vi "Save Digital Patterns.vi"(8 "error in (no error)":errorcluster, 10 "Patterns":T1[](array[typedef]), 11 "Item Ref in":T5 format="%.0x") -> (0 "error out":errorcluster)   [LabVIEW 2019, in "Engine Simulation Toolkit System Explorer.lvlib"]
uses:
  Engine Simulation Toolkit System Explorer.lvlib
  <vilib>/NI VeriStand/Custom Device API/Custom Device Item Ref.ctl
  Digital Pattern.ctl
  Digital Pattern Base.ctl
  Digital Pattern Remove Edge.ctl
  Digital Pattern Add Pulse.ctl
  Shared/Properties.vi
  <vilib>/NI VeriStand/Custom Device API/Set Item Property (String).vi
  <vilib>/NI VeriStand/Custom Device API/Set Item Property (Double).vi
  <vilib>/NI VeriStand/Custom Device API/Set Item Property (U16).vi
  <vilib>/NI VeriStand/Custom Device API/Set Item Property (Boolean).vi
  Shared/Engine Simulation Toolkit Shared.lvlib
  <vilib>/NI VeriStand/Custom Device API/Custom Device API.lvlib
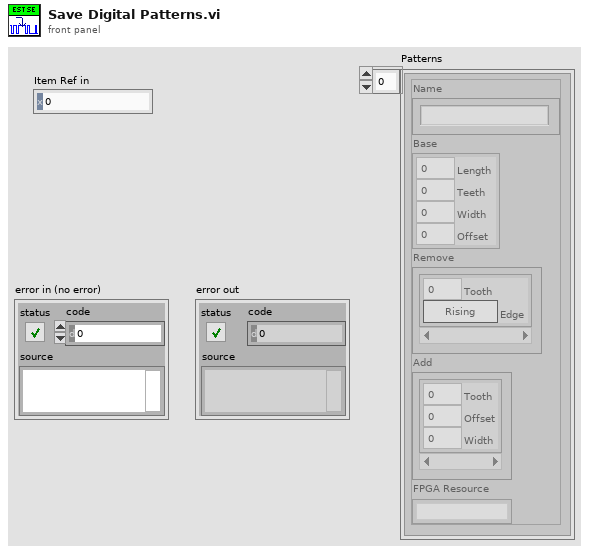
[diagram p1: front panel]
types:
  T1 = typedef "Engine Simulation Toolkit System Explorer.lvlib/Digital Pattern.ctl" = cluster{"Name":string, "Base":T2, "Remove":T3[], "Add":T4[], "FPGA Resource":string}
  T2 = typedef "Engine Simulation Toolkit System Explorer.lvlib/Digital Pattern Base.ctl" = cluster{"Length":dbl, "Teeth":u16, "Width":dbl, "Offset":dbl}
  T3 = typedef "Engine Simulation Toolkit System Explorer.lvlib/Digital Pattern Remove Edge.ctl" = cluster{"Tooth":u16, "Edge":bool}
  T4 = typedef "Engine Simulation Toolkit System Explorer.lvlib/Digital Pattern Add Pulse.ctl" = cluster{"Tooth":u16, "Offset":dbl, "Width":dbl}
  T5 = typedef "Custom Device API.lvlib/Custom Device Item Ref.ctl" = u64
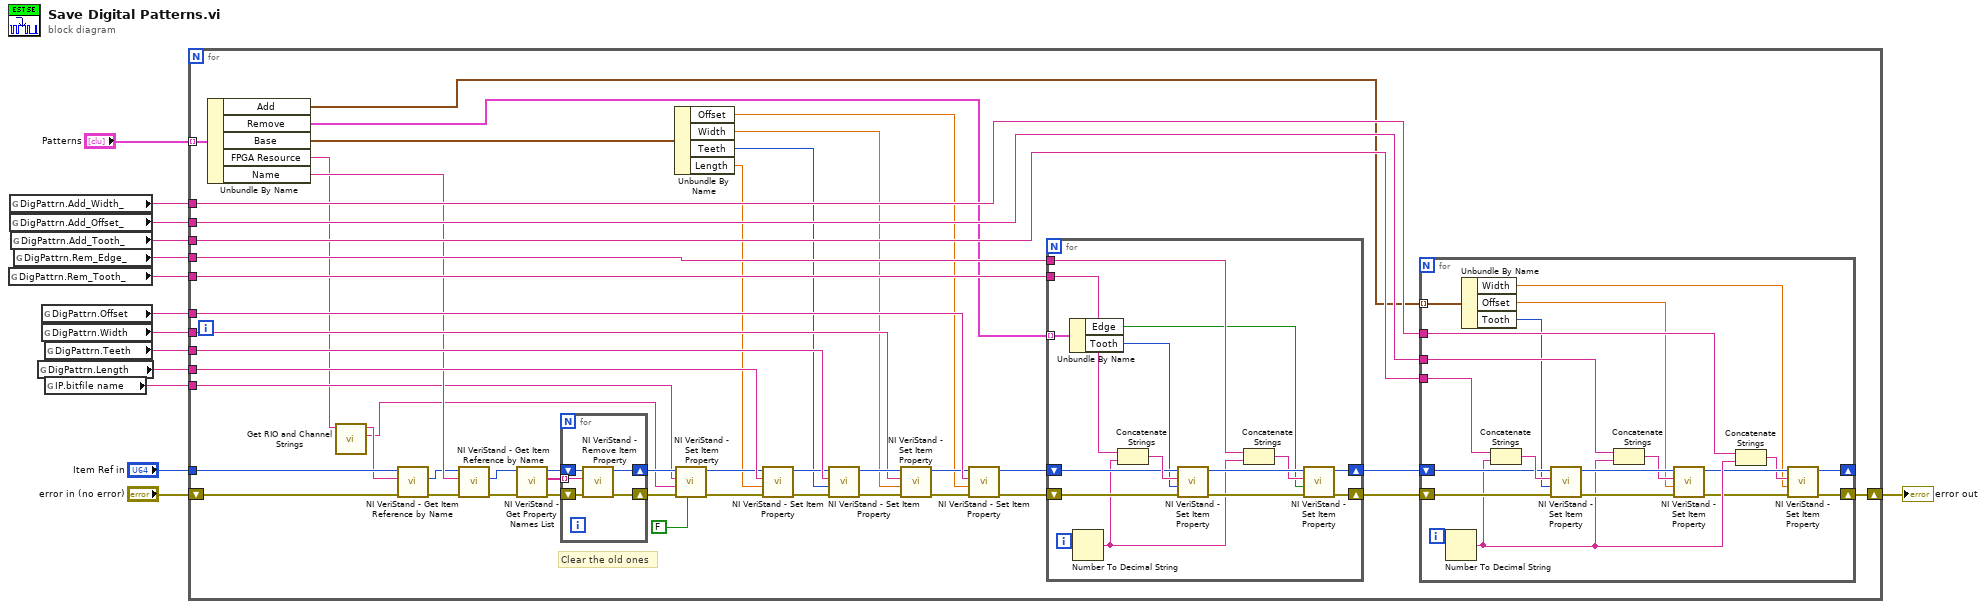
[diagram p0: block diagram]
diagram:
  n1 = global read "Properties.vi" "DigPattrn.Rem_Tooth_"() -> (w8:string)
  n2 = global read "Properties.vi" "DigPattrn.Add_Width_"() -> (w6:string)
  n3 = global read "Properties.vi" "DigPattrn.Add_Offset_"() -> (w5:string)
  n4 = global read "Properties.vi" "DigPattrn.Add_Tooth_"() -> (w4:string)
  n5 = global read "Properties.vi" "DigPattrn.Rem_Edge_"() -> (w7:string)
  n6 = global read "Properties.vi" "DigPattrn.Length"() -> (w12:string)
  n7 = global read "Properties.vi" "DigPattrn.Offset"() -> (w9:string)
  n8 = global read "Properties.vi" "DigPattrn.Width"() -> (w10:string)
  n9 = global read "Properties.vi" "DigPattrn.Teeth"() -> (w11:string)
  n10 = global read "Properties.vi" "IP.bitfile name"() -> (w1:string)
  n11 = for {
    shift-right: [w54] -> w13
    shift-left: "error in (no error)" -> [w20]
    tunnel: w12 -> [w61]
    tunnel: w11 -> [w60]
    tunnel: w10 -> [w43]
    tunnel: w9 -> [w59]
    tunnel: w8 -> [w58]
    tunnel: w7 -> [w57]
    tunnel: w4 -> [w55]
    tunnel: w5 -> [w42]
    tunnel: w6 -> [w56]
    tunnel: "Item Ref in" -> [w18]
    tunnel: "Patterns" -> [w41] mode=indexing
    tunnel: w1 -> [w29]
    # "Clear the old ones"
    n12 = Unbundle By Name(w41) -> ("Add"=w23:T4[], "Remove"=w24:T3[], "Base"=w38:T2, "FPGA Resource"=w16:string, "Name"=w39:string)
    n13 = call "Get RIO and Channel Strings.vi"("rio/channel"=w16) -> ("channel"=w15:string, "rio"=w17:string)  [unwired: 9 in]
    n14 = call <vilib>:"NI VeriStand - Get Item Reference by Name.vi"("error in (no error)"=w20, "Item Name"=w17, "Parent Ref in"=w18) -> ("error out"=w21:errorcluster, "Item Ref"=w19:T5)  [unwired: 5 in, 2 out]
    n15 = call <vilib>:"NI VeriStand - Get Item Reference by Name.vi"("error in (no error)"=w21, "Item Name"=w39, "Parent Ref in"=w19) -> ("error out"=w40:errorcluster, "Item Ref"=w36:T5)  [unwired: 5 in, 2 out]
    n16 = call <vilib>:"NI VeriStand - Get Property Names List.vi"("error in (no error)"=w40, "Item Ref in"=w36) -> ("error out"=w37:errorcluster, "Property Names"=w33:string[], "Item Ref out"=w34:T5)  [unwired: 7 in]
    n17 = for {
      tunnel: w33 -> [w97] mode=indexing
      shift-right: [w98] -> w31
      shift-left: w34 -> [w99]
      shift-right: [w100] -> w35
      shift-left: w37 -> [w101]
      n18 = call <vilib>:"NI VeriStand - Remove Item Property.vi"("error in (no error)"=w101, "Property Name"=w97, "Item Ref in"=w99) -> ("error out"=w100:errorcluster, "Item Ref out"=w98:T5)  [unwired: 6 in, 1 out]
    }
    n19 = Unbundle By Name(w38) -> ("Offset"=w25:dbl, "Width"=w26:dbl, "Teeth"=w27:u16, "Length"=w28:dbl)
    n20 = call-poly <vilib>:"NI VeriStand - Set Item Property.vi"("Binary String (T)"=FALSE, "error in (no error)"=w35, "Value"=w15, "Property Name"=w29, "Item Ref in"=w31) -> ("error out"=w32:errorcluster, "Item Ref out"=w30:T5)  [unwired: 4 in, 1 out]
    n21 = call-poly <vilib>:"NI VeriStand - Set Item Property.vi"("error in (no error)"=w32, "Value"=w28, "Property Name"=w61, "Item Ref in"=w30) -> ("error out"=w52:errorcluster, "Item Ref out"=w53:T5)  [unwired: 5 in, 1 out]
    n22 = call-poly <vilib>:"NI VeriStand - Set Item Property.vi"("error in (no error)"=w52, "Value"=w27, "Property Name"=w60, "Item Ref in"=w53) -> ("error out"=w50:errorcluster, "Item Ref out"=w51:T5)  [unwired: 5 in, 1 out]
    n23 = call-poly <vilib>:"NI VeriStand - Set Item Property.vi"("error in (no error)"=w50, "Value"=w26, "Property Name"=w43, "Item Ref in"=w51) -> ("error out"=w48:errorcluster, "Item Ref out"=w49:T5)  [unwired: 5 in, 1 out]
    n24 = call-poly <vilib>:"NI VeriStand - Set Item Property.vi"("error in (no error)"=w48, "Value"=w25, "Property Name"=w59, "Item Ref in"=w49) -> ("error out"=w44:errorcluster, "Item Ref out"=w45:T5)  [unwired: 5 in, 1 out]
    n25 = for {
      shift-right: [w86] -> w46
      shift-left: w44 -> [w94]
      shift-right: [w87] -> w47
      shift-left: w45 -> [w95]
      tunnel: w57 -> [w90]
      tunnel: w58 -> [w88]
      tunnel: w24 -> [w84] mode=indexing
      i -> [w93]
      n26 = Unbundle By Name(w84) -> ("Edge"=w82:bool, "Tooth"=w83:u16)
      n27 = Number To Decimal String(number=w93) -> (decimal integer string=w89:string)  [unwired: 1 in]
      n28 = Concatenate Strings(w88, w89) -> (w96:string)
      n29 = call-poly <vilib>:"NI VeriStand - Set Item Property.vi"("error in (no error)"=w94, "Value"=w83, "Property Name"=w96, "Item Ref in"=w95) -> ("error out"=w92:errorcluster, "Item Ref out"=w91:T5)  [unwired: 5 in, 1 out]
      n30 = Concatenate Strings(w90, w89) -> (w85:string)
      n31 = call-poly <vilib>:"NI VeriStand - Set Item Property.vi"("error in (no error)"=w92, "Value"=w82, "Property Name"=w85, "Item Ref in"=w91) -> ("error out"=w86:errorcluster, "Item Ref out"=w87:T5)  [unwired: 5 in, 1 out]
    }
    n32 = for {
      shift-right: [w71] -> w54
      shift-left: w46 -> [w79]
      shift-right: [w72] -> _
      shift-left: w47 -> [w80]
      tunnel: w42 -> [w75]
      tunnel: w55 -> [w73]
      tunnel: w56 -> [w70]
      tunnel: w23 -> [w65] mode=indexing
      i -> [w78]
      n33 = Number To Decimal String(number=w78) -> (decimal integer string=w74:string)  [unwired: 1 in]
      n34 = Unbundle By Name(w65) -> ("Width"=w62:dbl, "Offset"=w63:dbl, "Tooth"=w64:u16)
      n35 = Concatenate Strings(w73, w74) -> (w81:string)
      n36 = call-poly <vilib>:"NI VeriStand - Set Item Property.vi"("error in (no error)"=w79, "Value"=w64, "Property Name"=w81, "Item Ref in"=w80) -> ("error out"=w77:errorcluster, "Item Ref out"=w76:T5)  [unwired: 5 in, 1 out]
      n37 = Concatenate Strings(w75, w74) -> (w69:string)
      n38 = call-poly <vilib>:"NI VeriStand - Set Item Property.vi"("error in (no error)"=w77, "Value"=w63, "Property Name"=w69, "Item Ref in"=w76) -> ("error out"=w67:errorcluster, "Item Ref out"=w68:T5)  [unwired: 5 in, 1 out]
      n39 = Concatenate Strings(w70, w74) -> (w66:string)
      n40 = call-poly <vilib>:"NI VeriStand - Set Item Property.vi"("error in (no error)"=w67, "Value"=w62, "Property Name"=w66, "Item Ref in"=w68) -> ("error out"=w71:errorcluster, "Item Ref out"=w72:T5)  [unwired: 5 in, 1 out]
    }
  }
  "error out" <- w13
